vi "ImpulseResponse.vi"() -> ()   [LabVIEW 2015]
uses:
  <vilib>/express/express analysis/Spectral/Block/exnSpectralBlock spectral measurements RMS poly.vi
  <vilib>/express/express analysis/Spectral/Block/exnSpectralBlock spectral measurements RMS WFM.vi
  <vilib>/express/express analysis/Spectral/XNode/ExpressSpectralMeasurementsBlockNode.xnode
panel:
  in  "stop":bool
  in  "Averages":i32
  in  "Time":dbl
  in  "Rate":dbl
  out "Waveform Graph 2":cluster{"f0":dbl, "df":dbl, "magnitude":dbl[]}(graph)
  out "Waveform Graph":dbl[](graph)
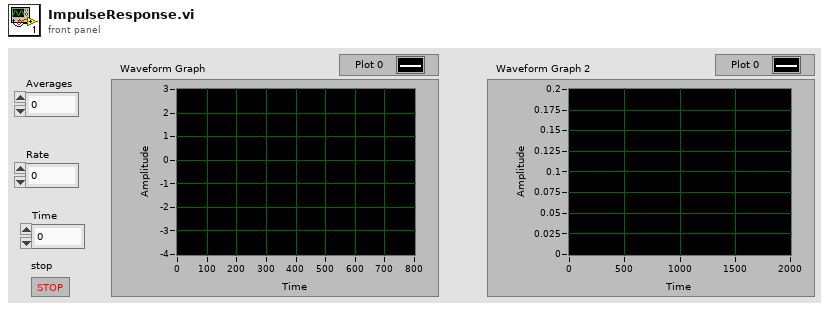
[diagram p1: front panel]
types:
  T1 = cluster{"averaging mode":u16, "weighting mode":u16, "number of averages":u32}
  T2 = cluster{"dB On (F)":bool, "unwrap phase (F)":bool, "convert to degree (F)":bool}
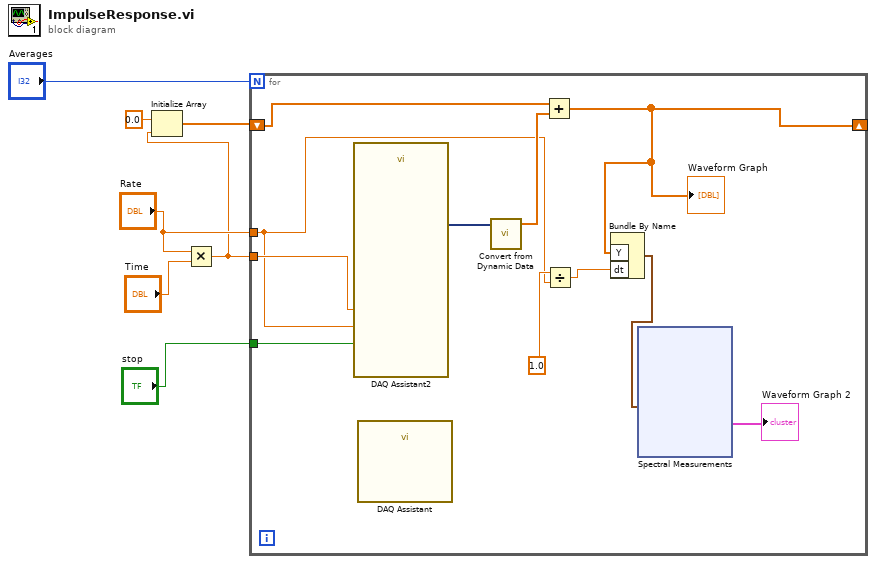
[diagram p0: block diagram]
diagram:
  n1 = Multiply(x="Rate", y="Time") -> (x*y=w1:dbl)
  n2 = Initialize Array(0.0 ("element"), w1) -> (w2:dbl[])
  n3 = for {
    N: "Averages" -> [_]
    tunnel: "stop" -> [w17]
    tunnel: w1 -> [w16]
    tunnel: "Rate" -> [w11]
    shift-right: [w13] -> _
    shift-left: w2 -> [w15]
    n4 = call "DAQ Assistant2"("rate"=w11, "number of samples"=w16, "stop (T)"=w17) -> ("data"=w18:dynamicdata)  [unwired: 14 in, 2 out]
    n5 = call "DAQ Assistant"() -> ()  [unwired: 18 in, 2 out]
    n6 = call "Convert from Dynamic Data"("Dynamic Data Type"=w18) -> ("Array"=w14:dbl[])  [unwired: 3 in]
    n7 = Add(x=w15, y=w14) -> (x+y=w13:dbl[])
    "Waveform Graph" <- w13
    n8 = Divide(x=1.0, y=w11) -> (x/y=w10:dbl)
    n9 = Bundle By Name("Y"=w13, "dt"=w10) -> (w9:waveform(dbl))  [unwired: 1 in]
    n10 = xnode "Spectral Measurements"("Signals"=w9) -> ("FFT - (RMS)"=→"Waveform Graph 2":cluster{"f0":dbl, "df":dbl, "magnitude":dbl[]})  [unwired: 1 in, 2 out]
  }
